vi "AB_Set_Preserve_Hierarchy.vi"(8 "error in (no error)":errorcluster, 9 "preserve hierarchy":bool, 10 "destination index":i32, 11 "destinations in":refnum<class "AB_Destination.lvclass">[](array[class])) -> (0 "error out":errorcluster, 3 "destinations out":refnum<class "AB_Destination.lvclass">[](array[class]))   [LabVIEW 2020]
uses:
  <vilib>/AppBuilder/AB_Classes/Destination/AB_Destination.lvclass
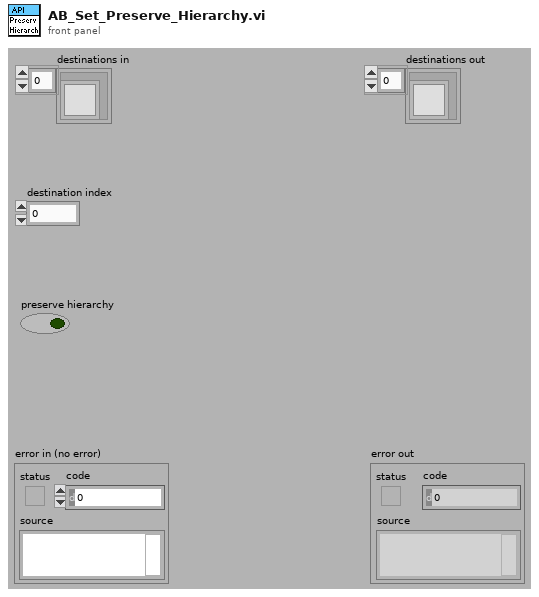
[diagram p1: front panel]
types:
  T1 = typedef "AB_Destination.ctl" = cluster{"destName":string, "path":path, "libraryName":string, "preserveHierarchy":bool, "eng_inBuild":bool, "eng_libraryReference":refnum<vi>, "eng_restictAddToNewLibrary":bool}
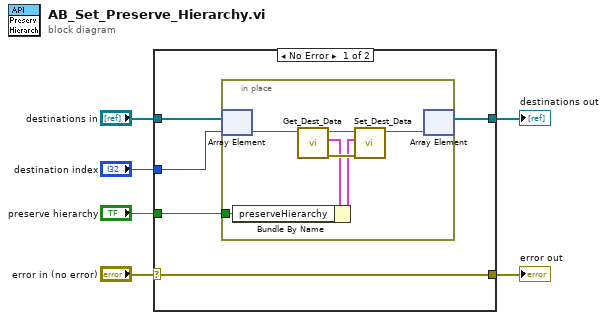
[diagram p0: block diagram]
diagram:
  n1 = case shown="No Error" "error in (no error)" {
    selector: "error in (no error)" -> [w9 w20]
    tunnel: [w9 w20] -> w5
    tunnel: "preserve hierarchy" -> [w11 _]
    tunnel: "destinations in" -> [w8 w19]
    tunnel: [w10 w19] -> w2
    tunnel: "destination index" -> [w7 _]
    frame No Error {
      n2 = in-place {
        in-place-border: w11 -> [w12]
        n3 = in-place-array #1(w8, w7) -> (w14:refnum<class "AB_Destination.lvclass">)
        n4 = call <vilib>:"Get_Dest_Data.vi"("Class in"=w14) -> ("error out"=w18:errorcluster, "destName"=w17:T1, "Class out"=w15:refnum<class "AB_Destination.lvclass">)  [unwired: 1 in, 7 out]
        n5 = Bundle By Name(cluster=w17, "preserveHierarchy"=w12) -> (w16:T1)
        n6 = call <vilib>:"Set_Dest_Data.vi"("error in (no error)"=w18, "destName"=w16, "Class in"=w15) -> ("Class out"=w13:refnum<class "AB_Destination.lvclass">)  [unwired: 8 out]
        n7 = in-place-array #1(w13) -> (w10:refnum<class "AB_Destination.lvclass">[])  [unwired: 1 out]
      }
    }
    frame Error {
    }
  }
  "error out" <- w5
  "destinations out" <- w2
